vi "USBImageWthFileOutputSUBVI.vi"(0 "Exposure Time (secs)":sgl format="%.2f") -> (1 "Vertical Binned Waveform Graph":i32[](graph), 2 "Intensity Graph":i32[][](graph))   [LabVIEW 2017]
uses:
  <vilib>/Utility/file.llb/Write Delimited Spreadsheet (DBL).vi
  atmcd32d.dll
panel:
  out "Status":u32
  out "Get Status":u32
  in  "Numeric":dbl
  out "Set Image":u32
  out "Set Gate Mode":u32
  out "Shut Down":u32
  out "Detector Y Pixels":i32
  out "Get Detector":u32
  out "Set Exposure Time":u32
  out "Set Trigger Mode":u32
  out "Set Readout Mode":u32
  out "Set Acquisition Mode":u32
  out "Check Timings":u32
  out "Detector X Pixels":i32
  out "Start Acquisition":u32
  out "Get Acquired Data":u32
  out "Calculated Exposure Value":sgl format="%.5f"
  out "Initialize":u32
  in  "Trigger":u32(ring) items=["Internal", "External"]
  # "Status"
  # "Return values"
  # "USB iStarIMAG32at.VI"
  # "Acquisition Mode: Single Scan\nReadout Mode: Full Resolution Image"
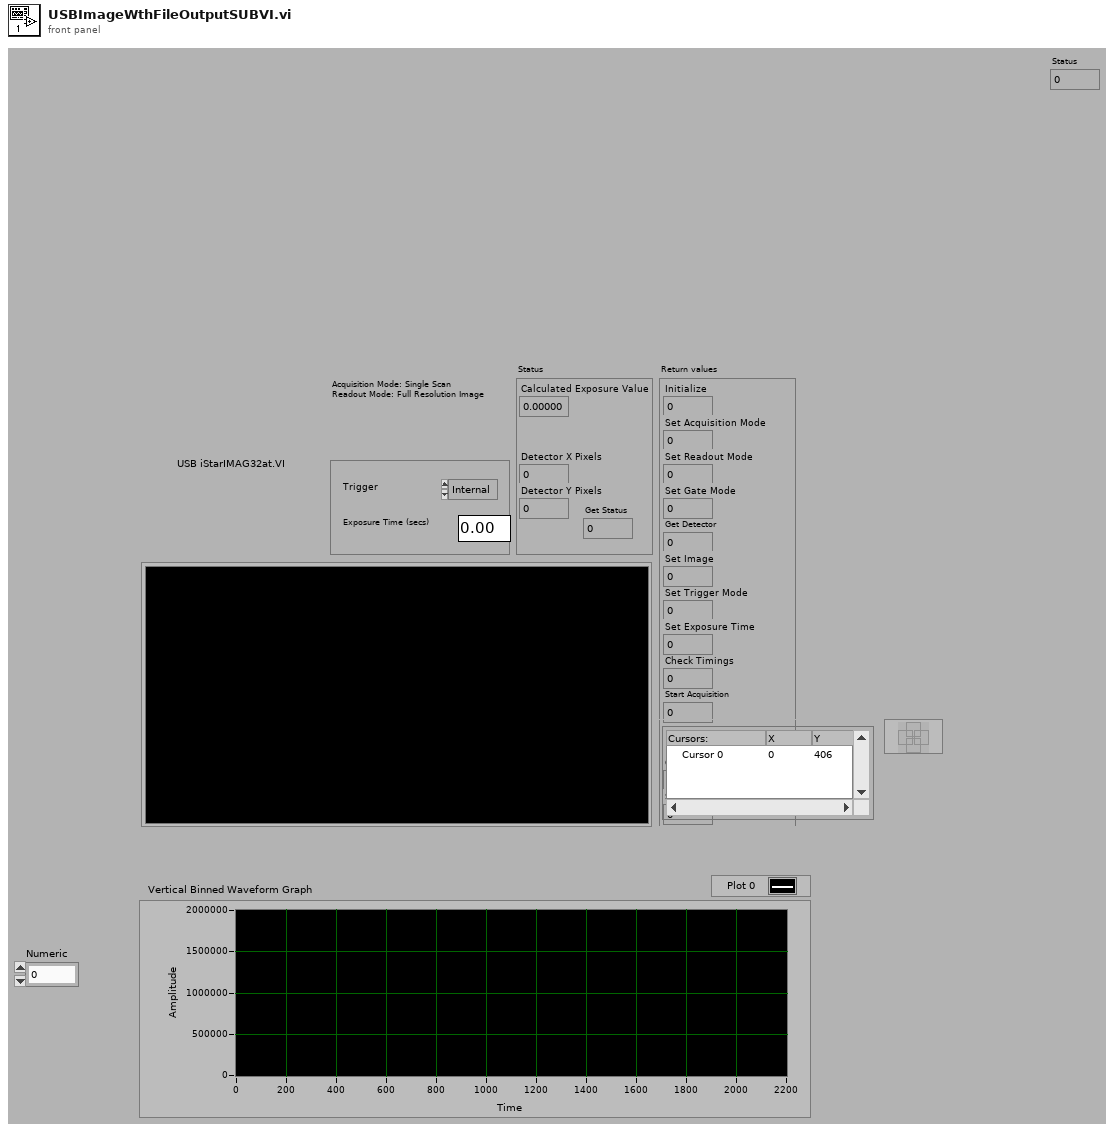
[diagram p1: front panel]
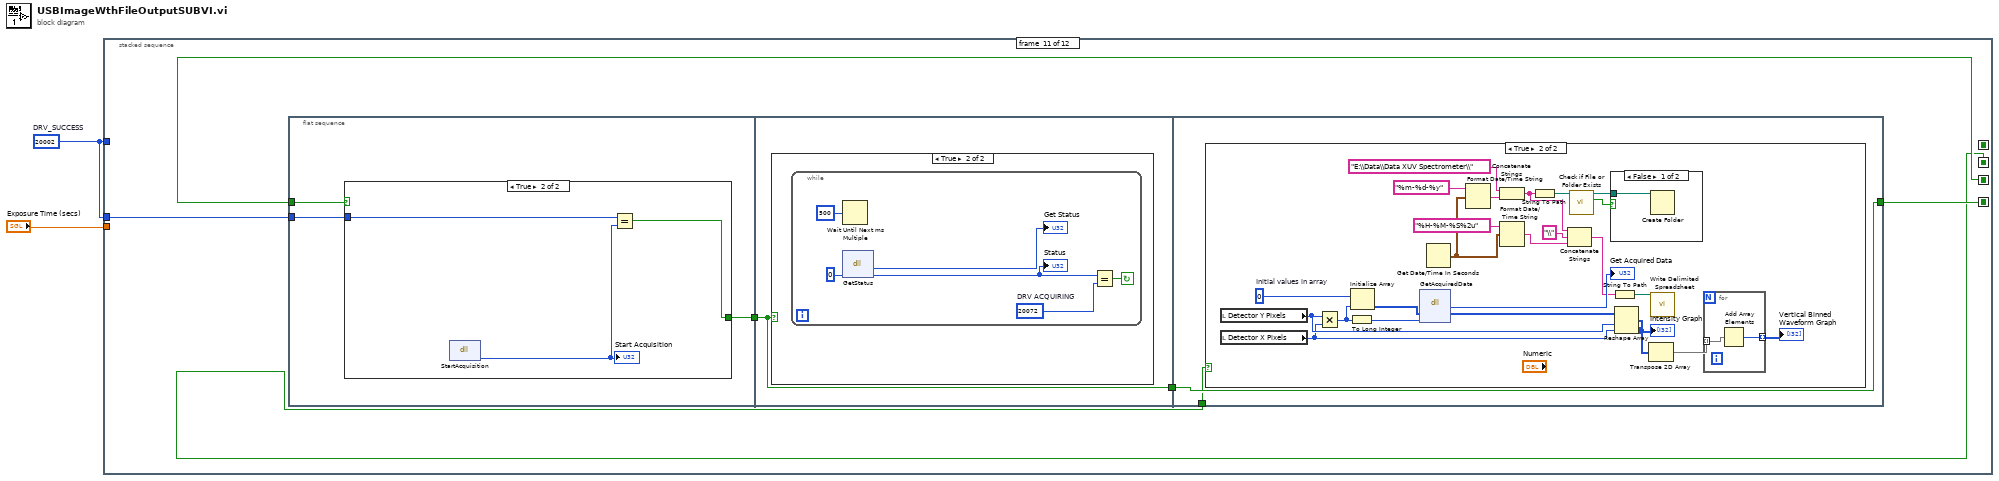
[diagram p0: block diagram]
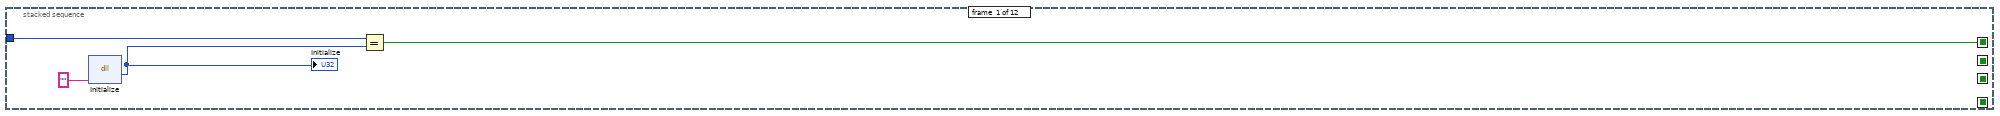
[diagram p2: hidden frame]
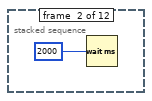
[diagram p3: hidden frame]
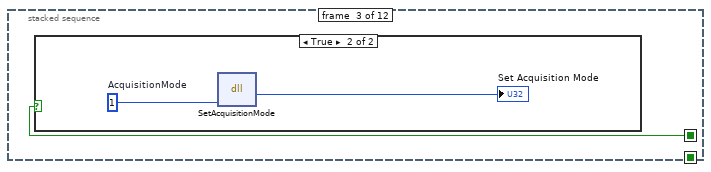
[diagram p4: hidden frame]
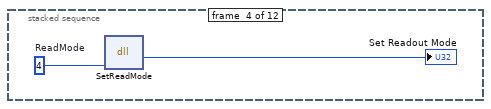
[diagram p6: hidden frame]
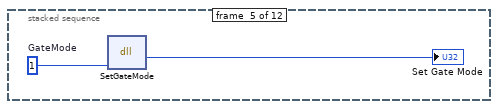
[diagram p7: hidden frame]
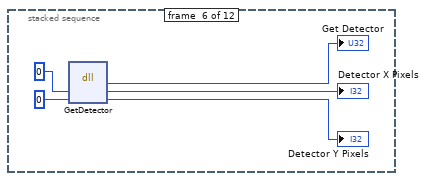
[diagram p8: hidden frame]
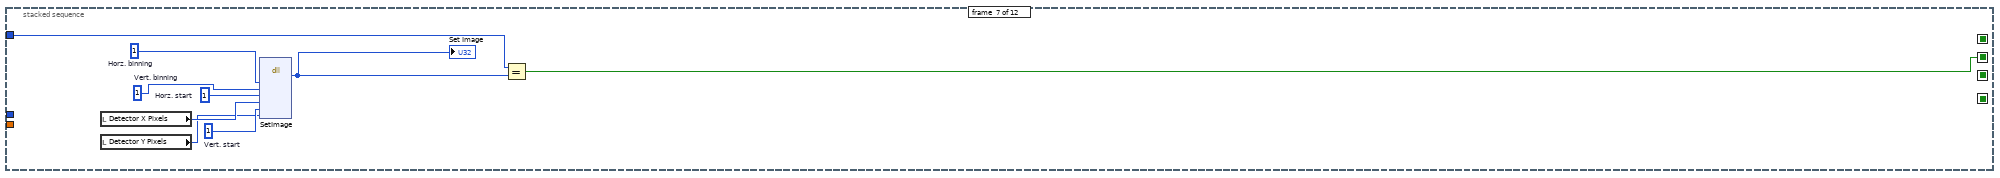
[diagram p9: hidden frame]
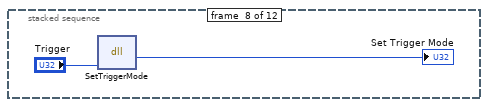
[diagram p10: hidden frame]
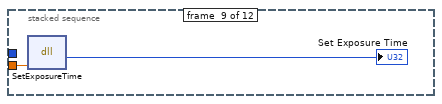
[diagram p11: hidden frame]
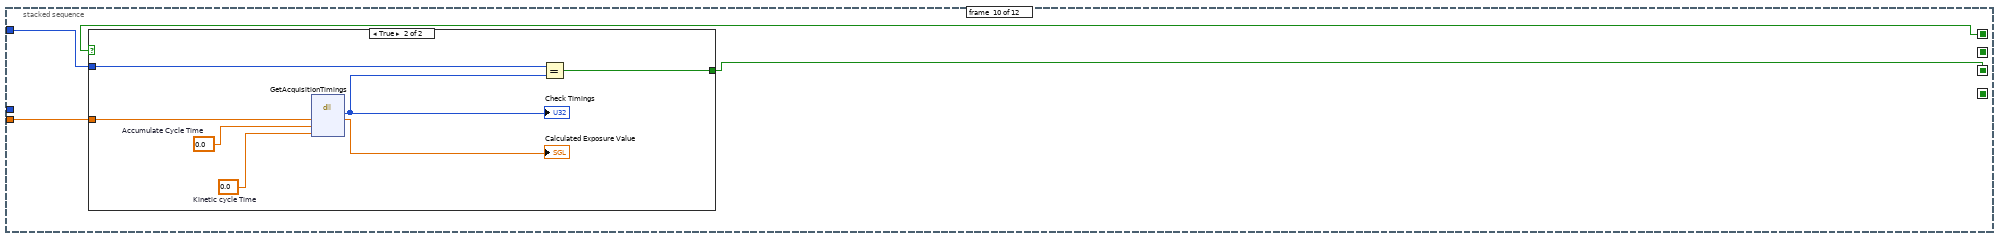
[diagram p12: hidden frame]
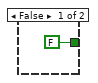
[diagram p13: hidden frame]
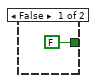
[diagram p14: hidden frame]
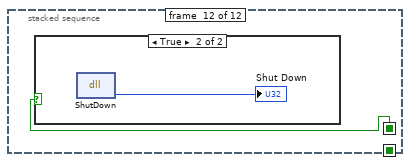
[diagram p18: hidden frame]
diagram:
  w1 = 20002  # DRV_SUCCESS
  n1 = stacked-sequence {
    seq-local: [w4 _ _ _ _ _ _ _ _ _ _ _] -> [_ _ w8 _ _ _ _ _ _ w33 _ w94]
    seq-local: [_ _ _ _ _ _ _ _ _ w34 _ _] -> [_ _ _ _ _ _ _ _ _ _ w50 _]
    seq-local: [_ _ _ _ _ _ _ _ _ _ w48 _] -> [_ _ _ _ _ _ _ _ _ _ _ _]
    seq-local: [_ _ _ _ _ _ w20 _ _ _ _ _] -> [_ _ _ _ _ _ _ _ _ _ w47 _]
    tunnel: "Exposure Time (secs)" -> [_ _ _ _ _ _ _ _ w32 w36 _ _]
    tunnel: w1 -> [w5 _ _ _ _ _ w22 _ _ w35 _ _]
    tunnel: w1 -> [_ _ _ _ _ _ _ _ _ _ w49 _]
    frame #0 {
      n2 = dll-call lib="atmcd32d.dll" fn="Initialize" label="Call Library Function Initialize"("") -> (w6:u32)  [unwired: 4 in, 2 out]
      "Initialize" <- w6
      n3 = Equal?(x=w5, y=w6) -> (x = y?=w4:bool)
    }
    frame #1 {
      n4 = Wait (ms)(milliseconds to wait=u32 2000) -> ()  [unwired: 1 out]
    }
    frame #2 {
      n5 = case shown="True" w8 {
        frame False {
        }
        frame True {
          w10 = u16 1  # AcquisitionMode
          n6 = dll-call lib="atmcd32d.dll" fn="SetAcquisitionMode" label="Call Library Function SetAcquisitionMode"(w10) -> (→"Set Acquisition Mode":u32)  [unwired: 4 in, 2 out]
        }
      }
    }
    frame #3 {
      w12 = u16 4  # ReadMode
      n7 = dll-call lib="atmcd32d.dll" fn="SetReadMode" label="Call Library Function SetReadMode"(w12) -> (→"Set Readout Mode":u32)  [unwired: 4 in, 2 out]
    }
    frame #4 {
      w14 = u16 1  # GateMode
      n8 = dll-call lib="atmcd32d.dll" fn="SetGateMode" label="Call Library Function SetGateMode"(w14) -> (→"Set Gate Mode":u32)  [unwired: 4 in, 2 out]
    }
    frame #5 {
      n9 = dll-call lib="atmcd32d.dll" fn="GetDetector" label="Call Library FunctionGetDetector"(i16 0, i16 0) -> (→"Get Detector":u32, →"Detector X Pixels":i32, →"Detector Y Pixels":i32)  [unwired: 3 in, 2 out]
    }
    frame #6 {
      w25 = u16 1  # Vert. start
      w26 = u16 1  # Horz. start
      w27 = u16 1  # Vert. binning
      w28 = u16 1  # Horz. binning
      n10 = local read "Detector X Pixels"() -> (w24:i32)
      n11 = local read "Detector Y Pixels"() -> (w23:i32)
      n12 = dll-call lib="atmcd32d.dll" fn="SetImage" label="Call Library Function SetImage"(w28, w27, w26, w24, w25, w23) -> (w21:u32)  [unwired: 9 in, 2 out]
      "Set Image" <- w21
      n13 = Equal?(x=w22, y=w21) -> (x = y?=w20:bool)
    }
    frame #7 {
      n14 = dll-call lib="atmcd32d.dll" fn="SetTriggerMode" label="Call Library Function SetTrigger Mode"("Trigger") -> (→"Set Trigger Mode":u32)  [unwired: 4 in, 2 out]
    }
    frame #8 {
      n15 = dll-call lib="atmcd32d.dll" fn="SetExposureTime" label="Call Library FunctionSet Exposure Time"(w32) -> (→"Set Exposure Time":u32)  [unwired: 4 in, 2 out]
    }
    frame #9 {
      n16 = case shown="True" w33 {
        tunnel: w36 -> [_ w41]
        tunnel: w35 -> [_ w38]
        tunnel: [FALSE w40] -> w34
        frame False {
        }
        frame True {
          w43 = sgl 0.0  # Accumulate Cycle Time
          w44 = sgl 0.0  # Kinetic cycle Time
          n17 = dll-call lib="atmcd32d.dll" fn="GetAcquisitionTimings" label="Call Library Function Check Timings"(w41, w43, w44) -> (w39:u32, →"Calculated Exposure Value":sgl)  [unwired: 5 in, 2 out]
          "Check Timings" <- w39
          n18 = Equal?(x=w38, y=w39) -> (x = y?=w40:bool)
        }
      }
    }
    frame #10 {
      n19 = flat-sequence {
        tunnel: w50 -> [w53]
        tunnel: w49 -> [w52]
        tunnel: [w51] -> w46
        tunnel: w46 -> [w58]
        tunnel: [w58] -> w45
        tunnel: [w66] -> w48
        tunnel: w45 -> [w66]
        tunnel: w47 -> [w65]
        frame #0 {
          n20 = case shown="True" w53 {
            tunnel: [FALSE w56] -> w51
            tunnel: w52 -> [_ w55]
            frame False {
            }
            frame True {
              n21 = dll-call lib="atmcd32d.dll" fn="StartAcquisition" label="Call Library Function start acquisition"() -> (w57:u32)  [unwired: 3 in, 2 out]
              "Start Acquisition" <- w57
              n22 = Equal?(x=w55, y=w57) -> (x = y?=w56:bool)
            }
          }
        }
        frame #1 {
          n23 = case shown="True" w58 {
            frame False {
            }
            frame True {
              n24 = while {
                stop <- w62 continue-if-true
                w61 = u16 20072  # DRV ACQUIRING
                n25 = Wait Until Next ms Multiple(millisecond multiple=u32 500) -> ()  [unwired: 1 out]
                n26 = dll-call lib="atmcd32d.dll" fn="GetStatus" label="Call Library Function GetAcquisitionStatus"(u16 0) -> (→"Get Status":u32, w60:u32)  [unwired: 3 in, 2 out]
                "Status" <- w60
                n27 = Equal?(x=w60, y=w61) -> (x = y?=w62:bool)
              }
            }
          }
        }
        frame #2 {
          n28 = case shown="True" w65 {
            frame False {
            }
            frame True {
              w90 = 0  # Initial values in array
              n29 = local read "Detector Y Pixels"() -> (w84:i32)
              n30 = local read "Detector X Pixels"() -> (w83:i32)
              n31 = Multiply(x=w84, y=w83) -> (x*y=w86:i32)
              n32 = To Long Integer(number=w86) -> (32bit integer=w87:i32)
              n33 = Initialize Array "Initialize Array"(w90, w86) -> (w88:i32[])
              n34 = dll-call lib="atmcd32d.dll" fn="GetAcquiredData" label="Call Library Function Get Acquired data"(w88, w87) -> (→"Get Acquired Data":u32, w85:i32[])  [unwired: 4 in, 2 out]
              n35 = Get Date/Time In Seconds() -> (seconds since 1Jan1904=w80:timestamp)
              n36 = Format Date/Time String(time format string (%c)="%m-%d-%y", seconds (now)=w80) -> (date/time string=w78:string)  [unwired: 1 in]
              n37 = Concatenate Strings("E:\\Data\\Data XUV Spectrometer\\" ("string"), w78) -> (w81:string)
              n38 = Format Date/Time String(time format string (%c)="%H-%M-%S%2u", seconds (now)=w80) -> (date/time string=w79:string)  [unwired: 1 in]
              n39 = String To Path(string=w81) -> (path=w77:path)
              n40 = Concatenate Strings(w81, "\\" ("string"), w79) -> (w82:string)
              n41 = call <vilib>:"Check if File or Folder Exists.vi"("path"=w77) -> ("file or folder exists?"=w75:bool, "dup path"=w76:path)  [unwired: 8 in, 1 out]
              n42 = case shown="False" w75 {
                tunnel: w76 -> [w93 _]
                frame False {
                  n43 = Create Folder(path (use dialog)=w93) -> ()  [unwired: 2 in, 3 out]
                }
                frame True {
                }
              }
              n44 = String To Path(string=w82) -> (path=w70:path)
              n45 = Reshape Array(w85, w84, w83) -> (w69:i32[][])
              "Intensity Graph" <- w69
              n46 = Transpose 2D Array(2D array=w69) -> (transposed array=w67:i32[][])
              n47 = call-poly <vilib>:"Write Delimited Spreadsheet.vi"("file path (dialog if empty)"=w70) -> ()  [unwired: 13 in, 2 out]
              n48 = for {
                tunnel: w67 -> [w92] mode=indexing
                tunnel: [w91] -> w68 mode=indexing
                n49 = Add Array Elements(numeric array=w92) -> (sum=w91:i32)
              }
              "Vertical Binned Waveform Graph" <- w68
            }
          }
        }
      }
    }
    frame #11 {
      n50 = case shown="True" w94 {
        frame False {
        }
        frame True {
          n51 = dll-call lib="atmcd32d.dll" fn="ShutDown" label="Call Library Function Shutdown"() -> (→"Shut Down":u32)  [unwired: 3 in, 2 out]
        }
      }
    }
  }
